vi "PickChannels.VI"(1 "# of channels?":u8=4, 2 "Channel":u8[](array[numeric])=[17, 18, 19, 20, 21, 22, 23, 24]) -> (0 "Command":string)   [LabVIEW 2021]
panel:
  # "Channel 1-16 represent single channels, while channel 17-24 are double channels, which are \ncombinations of channel 1-16"
  # "You are limited to 16 single or 8 double channels"
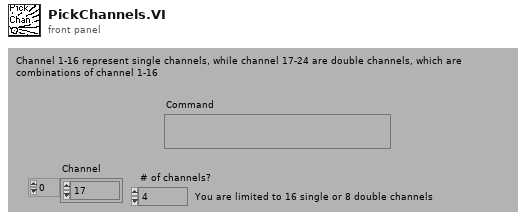
[diagram p1: front panel]
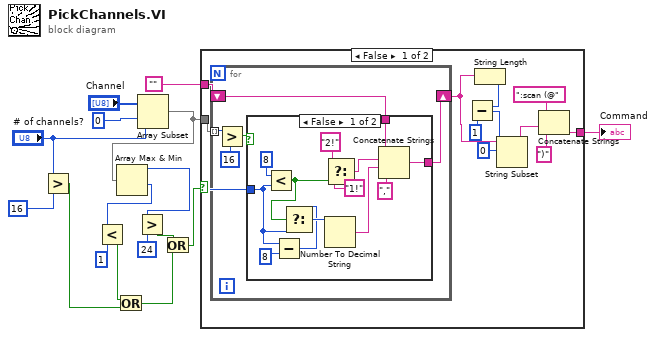
[diagram p0: block diagram]
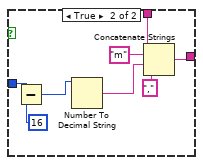
[diagram p2: hidden frame]
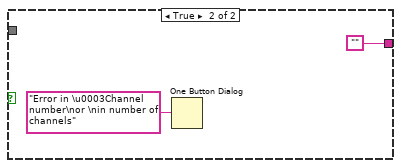
[diagram p3: hidden frame]
diagram:
  n1 = Greater?(x="# of channels?", y=16) -> (0:w4:bool)
  n2 = Array Subset(array="Channel", index=0, length="# of channels?") -> (w8:u8[])
  n3 = Array Max & Min(array=w8) -> (max value=w13:u8, min value=w12:u8)  [unwired: 2 out]
  n4 = Less?(x=w12, y=1) -> (x < y?=w3:bool)
  n5 = Or(x=w3, y=w4) -> (x .or. y?=w2:bool)
  n6 = Greater?(x=w13, y=24) -> (0:w10:bool)
  n7 = Or(x=w10, y=w2) -> (x .or. y?=w9:bool)
  n8 = case shown="False" w9 {
    tunnel: w8 -> [w27 _]
    tunnel: "" -> [w26 _]
    tunnel: [w17 ""] -> w14
    frame False {
      n9 = for {
        tunnel: w27 -> [w28] mode=indexing
        shift-right: [w32] -> w18
        shift-left: w26 -> [w31]
        n10 = Greater?(x=w28, y=16) -> (0:w29:bool)
        n11 = case shown="False" w29 {
          tunnel: [w36 w49] -> w32
          tunnel: w28 -> [w35 w48]
          tunnel: w31 -> [w33 w51]
          frame False {
            n12 = Less?(x=8, y=w35) -> (x < y?=w42:bool)
            n13 = Subtract(x=w35, y=8) -> (x-y=w44:i32)
            n14 = Select(t=w44, s=w42, f=w35) -> (s? t:f=w45:i32)
            n15 = Number To Decimal String(number=w45) -> (decimal integer string=w41:string)  [unwired: 1 in]
            n16 = Select(t="2!", s=w42, f="1!") -> (s? t:f=w38:string)
            n17 = Concatenate Strings(w33, w38, w41, ",") -> (w36:string)
          }
          frame True {
            n18 = Subtract(x=w48, y=16) -> (x-y=w46:i32)
            n19 = Number To Decimal String(number=w46) -> (decimal integer string=w53:string)  [unwired: 1 in]
            n20 = Concatenate Strings(w51, "m", w53, ",") -> (w49:string)
          }
        }
      }
      n21 = String Length(string=w18) -> (length=w24:i32)
      n22 = Subtract(x=w24, y=1) -> (x-y=w25:i32)
      n23 = String Subset(string=w18, offset (0)=0, length (rest)=w25) -> (substring=w21:string)
      n24 = Concatenate Strings(":scan (@", w21, ")") -> (w17:string)
    }
    frame True {
      n25 = One Button Dialog(message="Error in \u0003Channel number\nor \nin number of channels") -> ()  [unwired: 1 in, 1 out]
    }
  }
  "Command" <- w14
